vi "Acquire VISA Lock.vi"(8 "error in (no error)":errorcluster, 10 "timeout in ms (-1)":i32=-1, 11 "VISA resource name":refnum<visa-resource-name>) -> (0 "error out":errorcluster, 3 "VISA resource name out":refnum<visa-resource-name>)   [LabVIEW 2021, in "MB_VISA_Lock.lvlib"]
doc: "Attempts to acquire an exclusive lock on the session's VISA resource."
uses:
  <vilib>/Plasmionique/MB Master/MB_VISA_Lock/MB_VISA_Lock.lvlib
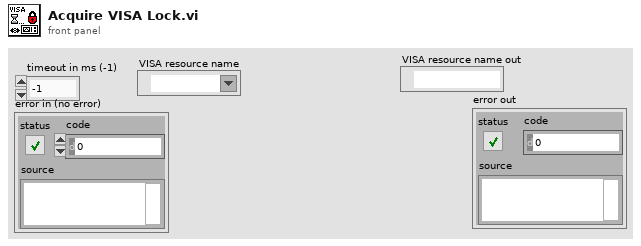
[diagram p1: front panel]
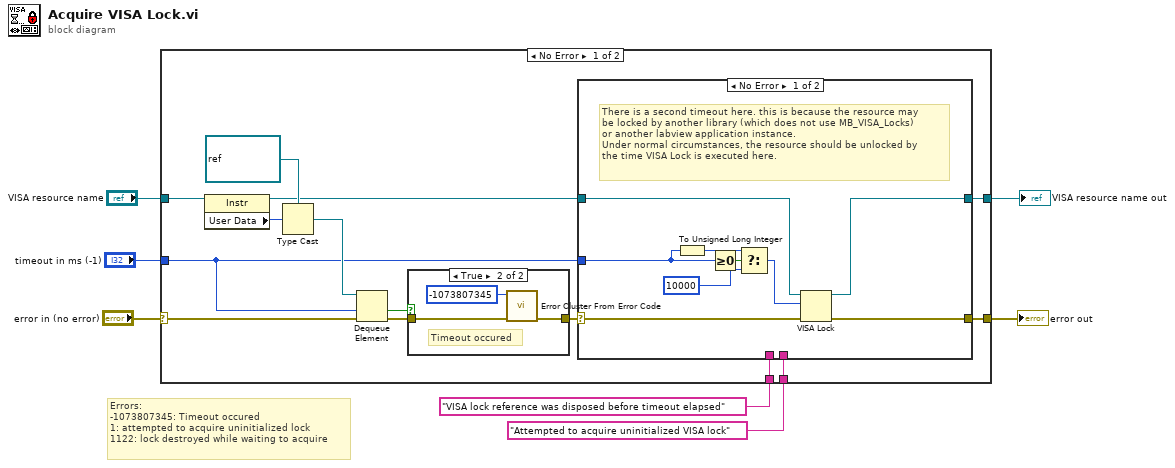
[diagram p0: block diagram]
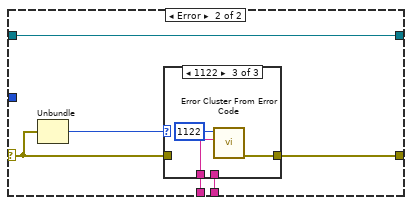
[diagram p2: hidden frame]
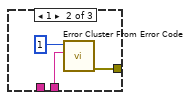
[diagram p4: hidden frame]
diagram:
  # "Errors:\n-1073807345: Timeout occured\n1: attempted to acquire uninitialized lock\n1122: lock destroyed while waiting to acquire"
  n1 = case shown="No Error" "error in (no error)" {
    selector: "error in (no error)" -> [w17 w48]
    tunnel: "timeout in ms (-1)" -> [w10 _]
    tunnel: [w13 w48] -> w6
    tunnel: [w12 w49] -> w5
    tunnel: "VISA resource name" -> [w21 w49]
    tunnel: "VISA lock reference was disposed before timeout elapsed" ("error message (\"\")") -> [w9 _]
    tunnel: "Attempted to acquire uninitialized VISA lock" ("error message (\"\")") -> [w8 _]
    frame No Error {
      n2 = property class="Instr"(reference=w21) -> (reference out=w11:refnum<visa-resource-name>, "User Data"=w20:u32)  [unwired: 1 in, 1 out]
      n3 = Type Cast(type=refnum<queue> refnum ("lock ref In"), x=w20) -> (*(type *) &x=w18:refnum<queue>)
      n4 = Dequeue Element(queue=w18, timeout in ms (-1)=w10, error in (no error)=w17) -> (timed out?=w16:bool, error out=w15:errorcluster)  [unwired: 2 out]
      n5 = case shown="True" w16 {
        tunnel: w15 -> [w44 w47]
        tunnel: [w44 w45] -> w14
        frame False {
        }
        frame True {
          # "Timeout occured"
          n6 = call <vilib>:"Error Cluster From Error Code.vi"("error in (no error)"=w47, "error code (0)"=-1073807345) -> ("error out"=w45:errorcluster)  [unwired: 7 in]
        }
      }
      n7 = case shown="No Error" w14 {
        selector: w14 -> [w30 w34]
        tunnel: [w29 w35] -> w13
        tunnel: [w28 w33] -> w12
        tunnel: w11 -> [w27 w33]
        tunnel: w10 -> [w26 _]
        tunnel: w9 -> [_ w32]
        tunnel: w8 -> [_ w31]
        frame No Error {
          # "There is a second timeout here. this is because the resource may\nbe locked by another library (which does not use MB_VISA_Locks)\nor another labview application instance.\nUnder normal circumstances, the resource should be unlocked by\nthe time VISA Lock is executed here."
          n8 = To Unsigned Long Integer(number=w26) -> (unsigned 32bit integer=w23:u32)
          n9 = Greater Or Equal To 0?(x=w26) -> (x >= 0?=w25:bool)
          n10 = Select(t=w23, s=w25, f=u32 10000 ("timeout (0)")) -> (s? t:f=w22:u32)
          n11 = VISA Lock(8:w30, 10:w22, 11:w27) -> (0:w29:errorcluster, 3:w28:refnum<visa-resource-name>)  [unwired: 2 in, 1 out]
        }
        frame Error {
          n12 = Unbundle(w34) -> ("code"=w36:i32)  [unwired: 2 out]
          n13 = case shown="1122" w36 {
            tunnel: w34 -> [w37 _ _]
            tunnel: [w37 w39 w42] -> w35
            tunnel: w32 -> [_ _ w41]
            tunnel: w31 -> [_ w38 _]
            frame 0, Default {
            }
            frame 1 {
              n14 = call <vilib>:"Error Cluster From Error Code.vi"("error message (\"\")"=w38, "error code (0)"=1) -> ("error out"=w39:errorcluster)  [unwired: 7 in]
            }
            frame 1122 {
              n15 = call <vilib>:"Error Cluster From Error Code.vi"("error message (\"\")"=w41, "error code (0)"=1122) -> ("error out"=w42:errorcluster)  [unwired: 7 in]
            }
          }
        }
      }
    }
    frame Error {
    }
  }
  "error out" <- w6
  "VISA resource name out" <- w5
